vi "fgv_4610_q.vi"(7 "cmd":T1, 8 "error in":errorcluster, 11 "action":T2) -> (0 "error out":errorcluster, 3 "queue out":refnum<queue>)   [LabVIEW 2019]
uses:
  _ctrl/BP4610_cmd.ctl
  _ctrl/create-rw-close.ctl
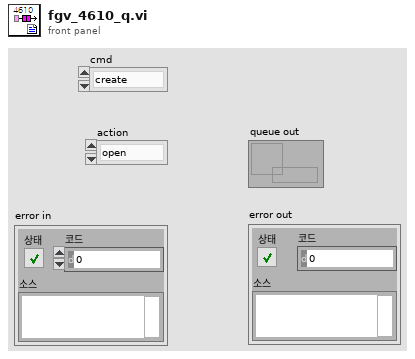
[diagram p1: front panel]
types:
  T1 = typedef "create-rw-close.ctl" = enum16{"create", "write", "read", "delete", "close"}
  T2 = typedef "BP4610_cmd.ctl" = enum16{"open", "read", "set", "set_seq", "limit", "limit_seq", "output on", "output off", "close"}
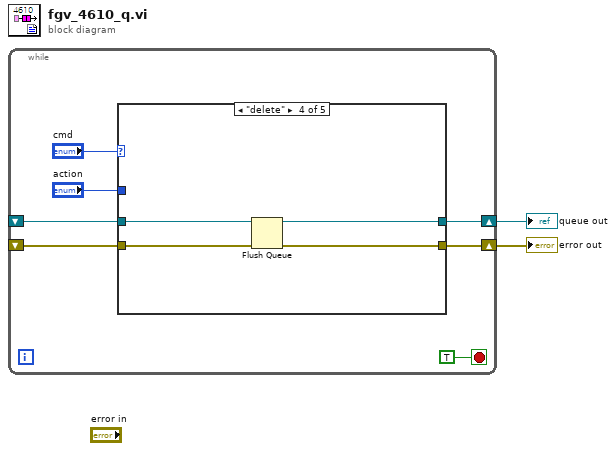
[diagram p0: block diagram]
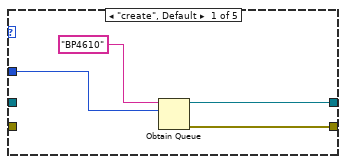
[diagram p2: hidden frame]
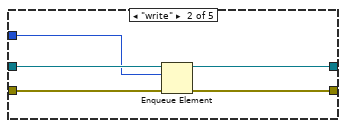
[diagram p3: hidden frame]
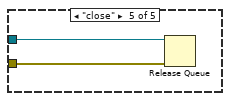
[diagram p5: hidden frame]
diagram:
  n1 = while {
    shift-right: [w4] -> w1
    shift-left: _ -> [w3]
    shift-right: [w5] -> w2
    shift-left: _ -> [w6]
    stop <- TRUE stop-if-true
    n2 = case shown="\"delete\"" "cmd" {
      tunnel: "action" -> [w13 w14 _ _ _]
      tunnel: w6 -> [_ w16 w20 w23 w26]
      tunnel: [w11 w15 w20 w21 _] -> w5
      tunnel: [w10 w17 w19 w22 _] -> w4
      tunnel: w3 -> [_ w18 w19 w24 w25]
      frame "create", Default {
        n3 = Obtain Queue(name (unnamed)="BP4610" ("이름(이름없음)"), element data type=w13) -> (queue out=w10:refnum<queue>, error out=w11:errorcluster)  [unwired: 3 in, 1 out]
      }
      frame "write" {
        n4 = Enqueue Element(queue=w18, element=w14, error in (no error)=w16) -> (queue out=w17:refnum<queue>, error out=w15:errorcluster)  [unwired: 1 in, 1 out]
      }
      frame "read" {
      }
      frame "delete" {
        n5 = Flush Queue(queue=w24, error in (no error)=w23) -> (queue out=w22:refnum<queue>, error out=w21:errorcluster)  [unwired: 1 out]
      }
      frame "close" {
        n6 = Release Queue(queue=w25, error in (no error)=w26) -> ()  [unwired: 1 in, 3 out]
      }
    }
  }
  "error out" <- w2
  "queue out" <- w1
